vi "Get Data.vi"(8 "error in (no error)":errorcluster, 10 "Expression in":string, 11 "Connection in":refnum<class "Connection.lvclass">) -> (0 "error out":errorcluster, 2 "Data out":refnum<class "Data.lvclass">, 3 "Connection out":refnum<class "Connection.lvclass">)   [LabVIEW 2012, in "MDSplus.lvlib" / "Connection.lvclass"]
uses:
  <vilib>/MDSplus/Classes/Connection_Class/Connection.lvclass
  <vilib>/MDSplus/Classes/Data_Class/Data.lvclass
  <vilib>/MDSplus/Classes/Connection_Class/Connection.lvclass/Connection.ctl
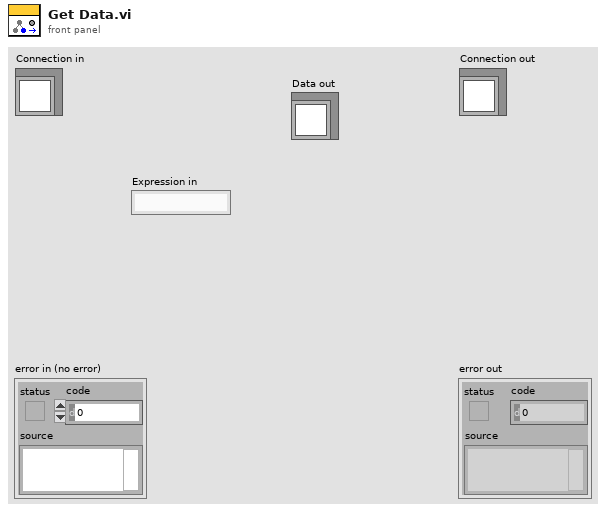
[diagram p1: front panel]
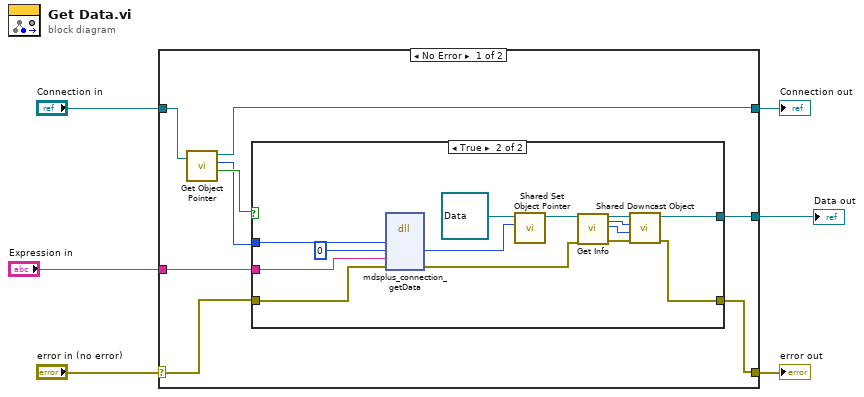
[diagram p0: block diagram]
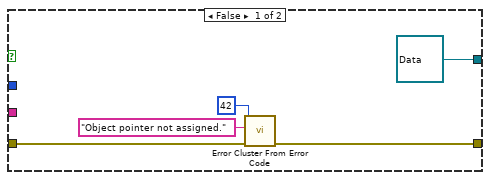
[diagram p2: hidden frame]
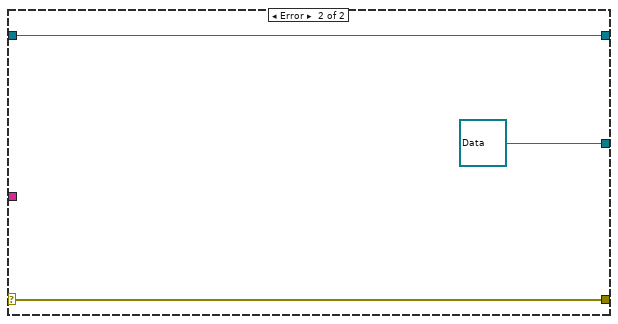
[diagram p3: hidden frame]
diagram:
  n1 = case shown="No Error" "error in (no error)" {
    selector: "error in (no error)" -> [w10 w36]
    tunnel: [w8 w36] -> w5
    tunnel: [w13 w35] -> w3
    tunnel: "Connection in" -> [w14 w35]
    tunnel: [w9 refnum<class "Data.lvclass"> refnum ("Data out")] -> w2
    tunnel: "Expression in" -> [w7 _]
    frame No Error {
      n2 = call <vilib>:"Get Object Pointer.vi"("Connection in"=w14) -> ("Assigned object pointer?"=w12:bool, "Object Pointer"=w11:i64, "Connection out"=w13:refnum<class "Connection.lvclass">)  [unwired: 7 in, 1 out]
      n3 = case shown="True" w12 {
        tunnel: [refnum<class "Data.lvclass"> refnum ("Data out") w25] -> w9
        tunnel: w11 -> [_ w24]
        tunnel: w10 -> [w16 w22]
        tunnel: [w15 w21] -> w8
        tunnel: w7 -> [_ w20]
        frame False {
          n4 = call <vilib>:"Error Cluster From Error Code.vi"("error in (no error)"=w16, "error message (\"\")"="Object pointer not assigned." ("error message (\"\")"), "error code (0)"=42) -> ("error out"=w15:errorcluster)  [unwired: 6 in]
        }
        frame True {
          n5 = dll-call lib="MDSobjectsLVShr" fn="mdsplus_connection_getData"("lvConnectionPtr"=w24, "lvDataPtrOut"=i64 0, "expressionIn"=w20, "error"=w22) -> ("lvDataPtrOut"=w31:i64, "error"=w23:errorcluster)  [unwired: 6 in, 2 out]
          n6 = call <vilib>:"Shared Set Object Pointer.vi"("Object Pointer"=w31, "Data in"=refnum<class "Data.lvclass"> refnum ("Data.lvclass")) -> ("Data out"=w30:refnum<class "Data.lvclass">)  [unwired: 9 in]
          n7 = call-dynamic "Get Info.vi"("Data in"=w30, "error in (no error)"=w23) -> ("Data out"=w29:refnum<class "Data.lvclass">, "Class type out"=w28:u8, "Data type out"=w27:u8, "error out"=w26:errorcluster)  [unwired: 12 in, 2 out]
          n8 = call <vilib>:"Shared Downcast Object.vi"("error in (no error)"=w26, "Data Type"=w27, "Class Type"=w28, "Data in"=w29) -> ("error out"=w21:errorcluster, "Data out"=w25:refnum<class "Data.lvclass">)  [unwired: 6 in]
        }
      }
    }
    frame Error {
    }
  }
  "error out" <- w5
  "Connection out" <- w3
  "Data out" <- w2
